vi "meter.vi"() -> ()   [LabVIEW 2019]
uses:
  <vilib>/Instr/_visa.llb/VISA Configure Serial Port (Instr).vi
panel:
  out "Strength":dbl(slide) scale=0.0..100.0
  out "Muscle Activity":i32(graph)
  in  "?":bool
  in  "Conect your Arduino and choose the COM port":refnum<visa-resource-name>
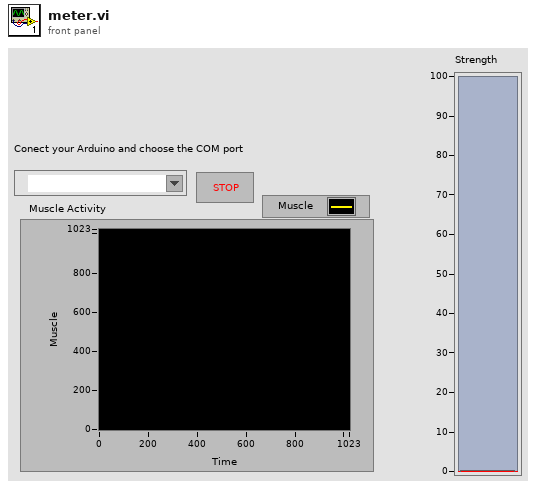
[diagram p1: front panel]
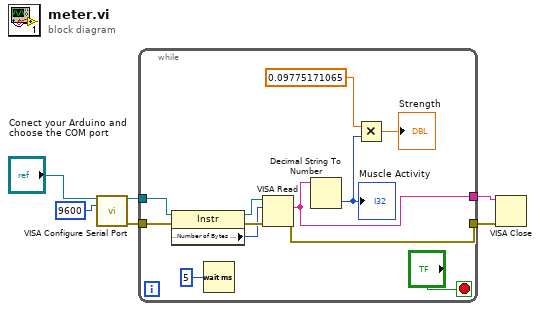
[diagram p0: block diagram]
diagram:
  n1 = call-poly "VISA Configure Serial Port"("VISA resource name"="Conect your Arduino and choose the COM port", "baud rate (9600)"=u32 9600) -> ("VISA resource name out"=w4:refnum<visa-resource-name>, "error out"=w3:errorcluster)  [unwired: 12 in]
  n2 = while {
    tunnel: w4 -> [w18]
    tunnel: w3 -> [w17]
    tunnel: [w16] -> w2
    tunnel: [w7] -> w1
    stop <- "?" stop-if-true
    n3 = property class="Instr"(reference=w18, error in=w17) -> (reference out=w15:refnum<visa-resource-name>, error out=w14:errorcluster, "Serial Settings:Number of Bytes at Serial Port"=w13:u32)
    n4 = Wait (ms)(milliseconds to wait=u32 5) -> ()  [unwired: 1 out]
    n5 = VISA Read(VISA resource name=w15, byte count=w13, error in (no error)=w14) -> (read buffer=w7:string, error out=w16:errorcluster)  [unwired: 2 out]
    n6 = Decimal String To Number(string=w7) -> (number=w9:i32)  [unwired: 2 in, 1 out]
    "Muscle Activity" <- w9
    n7 = Multiply(x=0.09775171065, y=w9) -> (x*y=→"Strength":dbl)
  }
  n8 = VISA Close(VISA resource name=w1, error in (no error)=w2) -> ()  [unwired: 1 out]
